vi "Write Vector Network Analyzer.lvclass.vi"(10 "Vector Network Analyzer.lvclass":refnum<class "Vector Network Analyzer.lvclass">, 11 "S Parameter in":refnum<class "S Parameter.lvclass">) -> (3 "S Parameter out":refnum<class "S Parameter.lvclass">)   [LabVIEW 2020, in "S Parameter.lvclass"]
uses:
  S Parameter.lvclass
  Instruments/Vector Network Analyzer/Vector Network Analyzer.lvclass
  S Parameter.lvclass/S Parameter.ctl
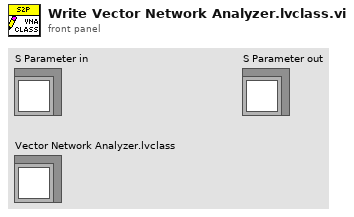
[diagram p1: front panel]
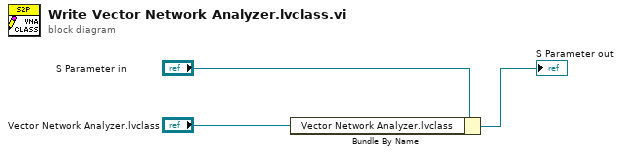
[diagram p0: block diagram]
diagram:
  n1 = Bundle By Name(cluster="S Parameter in", "Vector Network Analyzer.lvclass"="Vector Network Analyzer.lvclass") -> (→"S Parameter out":refnum<class "S Parameter.lvclass">)
